vi "Serialize Byte Array.vi"(3 "data":u8[](array[numeric])) -> (1 "bytes":u8[](array[numeric]))   [LabVIEW 2020, in "NI_SFTP.lvlib" / "Low Level Connection.lvclass"]
uses:
  <vilib>/net/SFTP/Low Level Connection/Low Level Connection.lvclass
  d3fa6884-f613-3fef-0085-967f4ca98a3f.vi
  d3fa6884-f613-3fef-0085-967f4ca98a3f.vi/23199ad8-9c00-3fe8-00d7-de5c3ecebd3f.vi
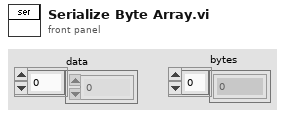
[diagram p1: front panel]
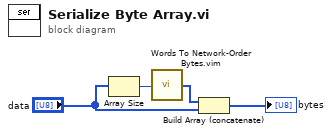
[diagram p0: block diagram]
diagram:
  n1 = Array Size(array="data") -> (size(s)=w1:i32)
  n2 = call "Words To Network-Order Bytes.vim"("word"=w1) -> ("bytes"=w2:u8[])
  n3 = Build Array (concatenate)(w2, "data") -> (→"bytes":u8[])
